vi "init.vi"(8 "error in (no error)":errorcluster, 9 "Samples To Average":i32, 10 "+5VA Channel":refnum<k21>, 11 "ConvertDACRawToEngStrategy in":refnum<class "ConvertDACRawToEngStrategy.lvclass">) -> (0 "error out":errorcluster, 3 "ConvertDACRawToEngStrategy out":refnum<class "ConvertDACRawToEngStrategy.lvclass">)   [LabVIEW 2015, in "ConvertDACRawToEngStrategy.lvclass"]
uses:
  ConvertDACRawToEngStrategy.lvclass
  ConvertDACRawToEngStrategy.lvclass/ConvertDACRawToEngStrategy.ctl
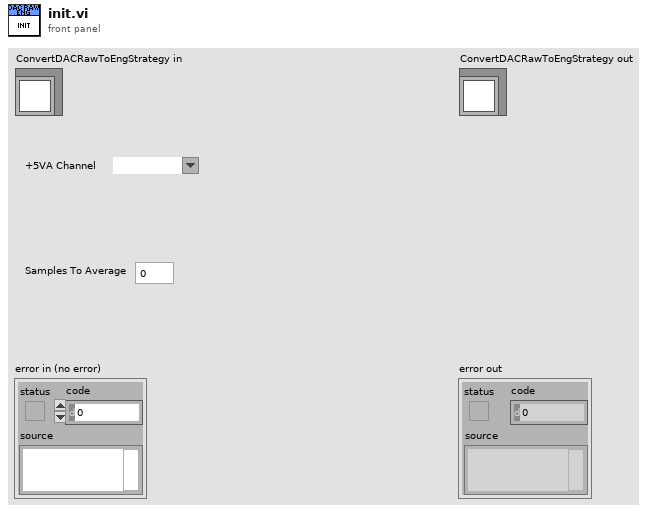
[diagram p1: front panel]
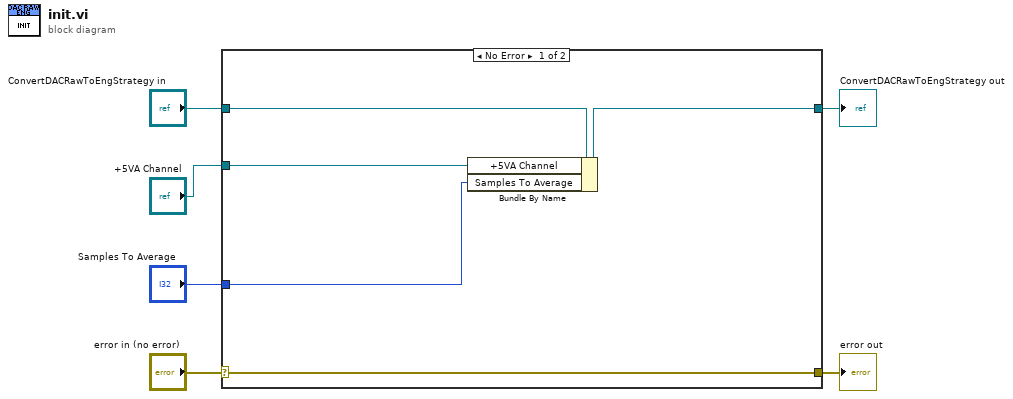
[diagram p0: block diagram]
diagram:
  n1 = case shown="No Error" "error in (no error)" {
    selector: "error in (no error)" -> [w11 w13]
    tunnel: [w11 w13] -> w5
    tunnel: [w7 w12] -> w3
    tunnel: "ConvertDACRawToEngStrategy in" -> [w8 w12]
    tunnel: "+5VA Channel" -> [w10 _]
    tunnel: "Samples To Average" -> [w9 _]
    frame No Error {
      n2 = Bundle By Name(cluster=w8, "+5VA Channel"=w10, "Samples To Average"=w9) -> (w7:refnum<class "ConvertDACRawToEngStrategy.lvclass">)
    }
    frame Error {
    }
  }
  "error out" <- w5
  "ConvertDACRawToEngStrategy out" <- w3
